vi "Core-Wait.vi"(8 "error in (no error)":errorcluster, 11 "Engine in":refnum<class "Engine.lvclass">) -> (0 "error out":errorcluster, 3 "Engine out":refnum<class "Engine.lvclass">)   [LabVIEW 2024, in "GLF.lvlib" / "Engine.lvclass"]
uses:
  Engine.lvclass
  Engine.lvclass/Engine.ctl
  <vilib>/Saukko/LV SDL3/Sources/SDL3/Timer/Timer.lvlib
  6955d516-8360-42b9-bfaf-a0de5a30dce7.vi
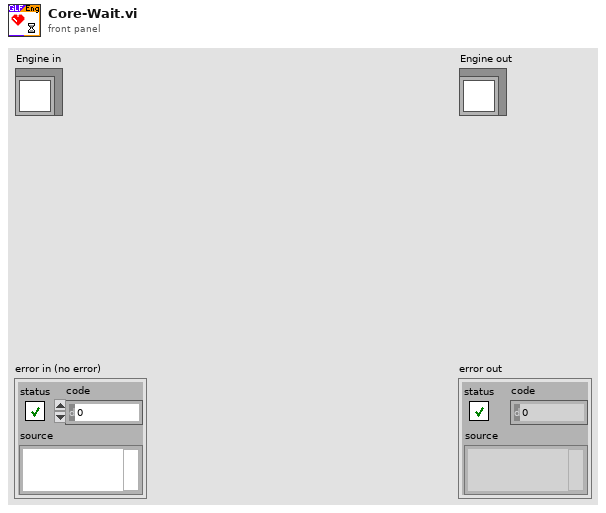
[diagram p1: front panel]
types:
  T1 = typedef "GLF.lvlib/Engine.lvclass/DVR--cluster.ctl" = cluster{"CMD Queue":T2, "Config":T3, "Ctxt":T5, "Metrics":T6}
  T2 = typedef "GLF.lvlib/Engine.lvclass/Command--queue.ctl" = refnum<queue>
  T3 = typedef "GLF.lvlib/Engine.lvclass/Config--cluster.ctl" = cluster{"Quit On Last Window Closed":bool, "VSync":T4, "FPS Target":dbl}
  T4 = typedef "GLF.lvlib/Engine.lvclass/VSync--enum.ctl" = enum16{"Disabled", "Enabled", "Adaptative"}
  T5 = typedef "GLF.lvlib/Engine.lvclass/Context--cluster.ctl" = cluster{"Ticks Begin":u64, "VSync Enabled":bool}
  T6 = typedef "GLF.lvlib/Engine.lvclass/Metrics--cluster.ctl" = cluster{"Uptime [ms]":u64, "Loop Time [ms]":u64}
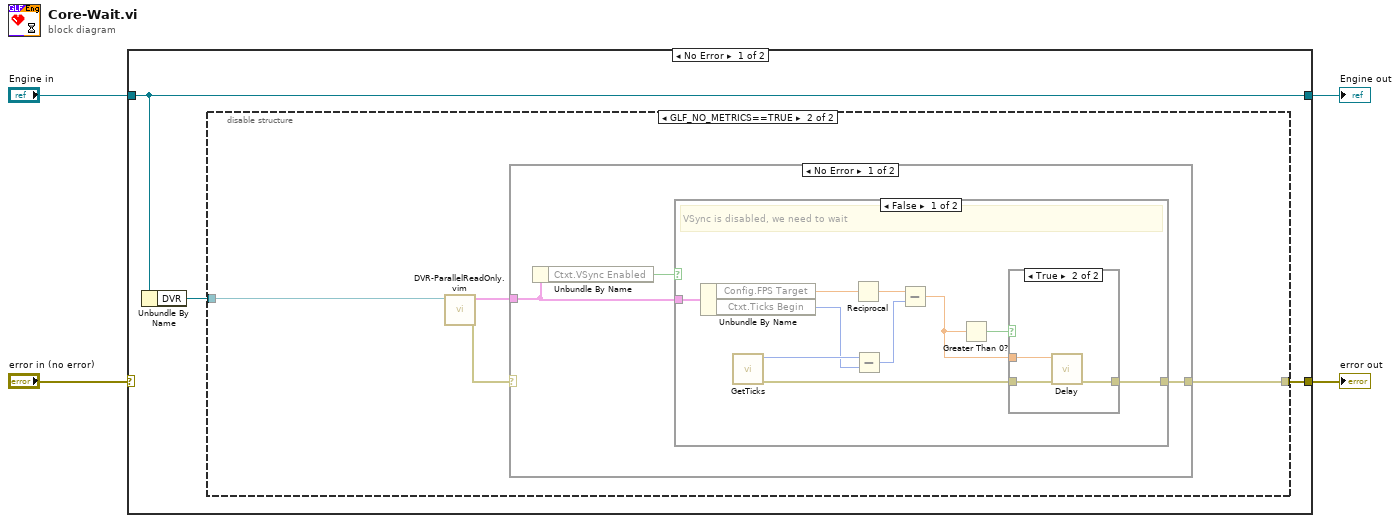
[diagram p0: block diagram]
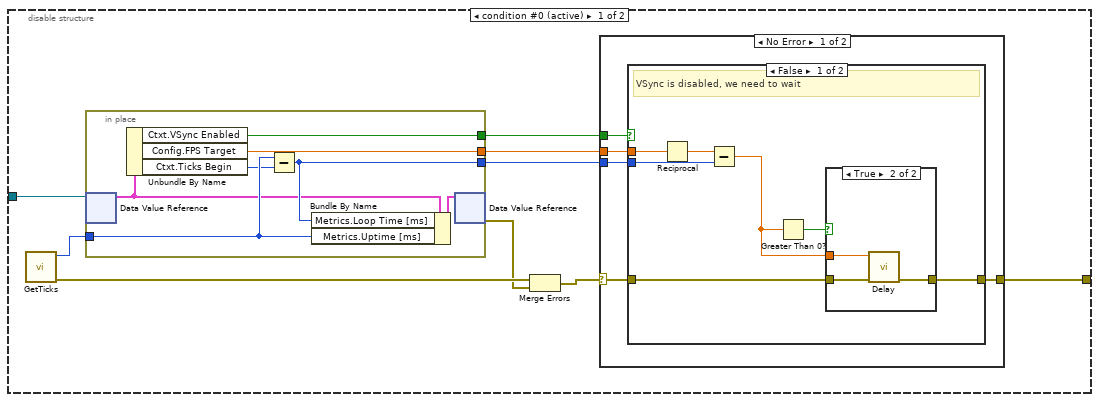
[diagram p2: hidden frame]
diagram:
  n1 = case shown="No Error" "error in (no error)" {
    selector: "error in (no error)" -> [_ w64]
    tunnel: [w6 w64] -> w4
    tunnel: "Engine in" -> [w7 w65]
    tunnel: [w7 w65] -> w1
    frame No Error {
      n2 = Unbundle By Name(w7) -> ("DVR"=w5:refnum<data-value>)
      n3 = disable-structure shown="GLF_NO_METRICS==TRUE" {
        disable-tunnel: [w16 w45] -> w6
        disable-tunnel: w5 -> [w15 w44]
        frame condition #0 (active) {
          n4 = call <vilib>:"GetTicks.vi"() -> ("error out"=w10:errorcluster, "Ticks [ms]"=w14:u64)  [unwired: 10 in]
          n5 = in-place {
            in-place-border: w14 -> [w40]
            in-place-border: [w39] -> w13
            in-place-border: [w37] -> w12
            in-place-border: [w36] -> w11
            n6 = in-place-dvr #1(w15) -> (w38:T1)  [unwired: 1 out]
            n7 = Unbundle By Name(w38) -> ("Ctxt.VSync Enabled"=w37:bool, "Config.FPS Target"=w36:dbl, "Ctxt.Ticks Begin"=w35:u64)
            n8 = Subtract(x=w40, y=w35) -> (x-y=w39:u64)
            n9 = Bundle By Name(cluster=w38, "Metrics.Loop Time [ms]"=w39, "Metrics.Uptime [ms]"=w40) -> (w41:T1)
            n10 = in-place-dvr #1(w41) -> (w8:errorcluster)  [unwired: 1 out]
          }
          n11 = Merge Errors(w10, w8) -> (w9:errorcluster)
          n12 = case shown="No Error" w9 {
            selector: w9 -> [w17 w34]
            tunnel: [w21 w34] -> w16
            tunnel: w13 -> [w20 _]
            tunnel: w12 -> [w19 _]
            tunnel: w11 -> [w18 _]
            frame No Error {
              n13 = case shown="False" w19 {
                tunnel: w17 -> [w24 w33]
                tunnel: [w27 w33] -> w21
                tunnel: w20 -> [w22 _]
                tunnel: w18 -> [w23 _]
                frame False {
                  # "VSync is disabled, we need to wait"
                  n14 = Reciprocal(x=w23) -> (1/x=w28:dbl)
                  n15 = Subtract(x=w28, y=w22) -> (x-y=w26:dbl)
                  n16 = Greater Than 0?(x=w26) -> (x > 0?=w25:bool)
                  n17 = case shown="True" w25 {
                    tunnel: w24 -> [w29 w32]
                    tunnel: [w29 w31] -> w27
                    tunnel: w26 -> [_ w30]
                    frame False {
                    }
                    frame True {
                      n18 = call <vilib>:"Delay.vi"("No Error"=w32, "ms"=w30) -> ("error out"=w31:errorcluster)  [unwired: 9 in]
                    }
                  }
                }
                frame True {
                  # "No need to wait, this is done with the render present function"
                }
              }
            }
            frame Error {
            }
          }
        }
        frame condition #1 {
          n19 = call "DVR-ParallelReadOnly.vim"("DVR"=w44) -> ("Error Out"=w43:errorcluster, "Data"=w42:T1)  [unwired: 9 in]
          n20 = case shown="No Error" w43 {
            selector: w43 -> [_ w63]
            tunnel: [w47 w63] -> w45
            tunnel: w42 -> [w46 _]
            frame No Error {
              n21 = Unbundle By Name(w46) -> ("Ctxt.VSync Enabled"=w48:bool)
              n22 = case shown="False" w48 {
                tunnel: [w56 _] -> w47
                tunnel: w46 -> [w53 _]
                frame False {
                  # "VSync is disabled, we need to wait"
                  n23 = Unbundle By Name(w53) -> ("Config.FPS Target"=w58:dbl, "Ctxt.Ticks Begin"=w50:u64)
                  n24 = call <vilib>:"GetTicks.vi"() -> ("error out"=w52:errorcluster, "Ticks [ms]"=w51:u64)  [unwired: 10 in]
                  n25 = Reciprocal(x=w58) -> (1/x=w57:dbl)
                  n26 = Subtract(x=w51, y=w50) -> (x-y=w49:u64)
                  n27 = Subtract(x=w57, y=w49) -> (x-y=w55:dbl)
                  n28 = Greater Than 0?(x=w55) -> (x > 0?=w54:bool)
                  n29 = case shown="True" w54 {
                    tunnel: w52 -> [w59 w62]
                    tunnel: [w59 w61] -> w56
                    tunnel: w55 -> [_ w60]
                    frame False {
                    }
                    frame True {
                      n30 = call <vilib>:"Delay.vi"("No Error"=w62, "ms"=w60) -> ("error out"=w61:errorcluster)  [unwired: 9 in]
                    }
                  }
                }
                frame True {
                  # "No need to wait, this is done with the render present function"
                }
              }
            }
            frame Error {
            }
          }
        }
      }
    }
    frame Error {
    }
  }
  "error out" <- w4
  "Engine out" <- w1
